vi "NI VeriStand - Close Model Manager Reference.vi"(8 "error in (no error)":errorcluster, 11 "ModelManager":T1) -> (0 "error out":errorcluster)   [LabVIEW 2020, in "NI_VS ModelManager ExecutionAPI.lvlib"]
doc: "Closes an open reference to the model manager on the VeriStand Gateway. Use this VI to close each model manager reference that you open with the Open Model Manager Reference VI."
uses:
  <vilib>/NI VeriStand/Execution/ModelManager/NI_VS ModelManager ExecutionAPI.lvlib
  <vilib>/NI VeriStand/Execution/ModelManager/ModelManagerAPI.ctl
  NationalInstruments.VeriStand.ClientAPI
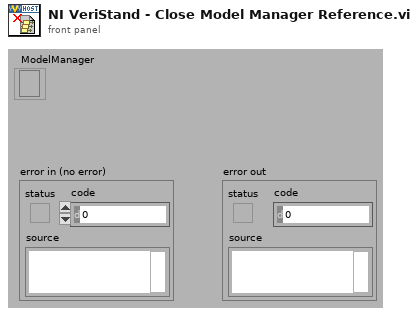
[diagram p1: front panel]
types:
  T1 = typedef "NI_VS ModelManager ExecutionAPI.lvlib/ModelManagerAPI.ctl" = refnum<k24>
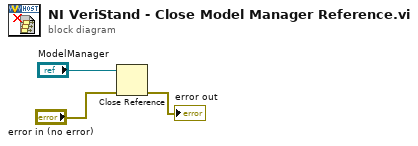
[diagram p0: block diagram]
diagram:
  n1 = Close Reference(reference="ModelManager", error in (no error)="error in (no error)") -> (error out=→"error out":errorcluster)
